vi "Update SequencerInfo.vi"(8 "error in (no error)":errorcluster, 10 "SequencerInfo":refnum<class "SequencerInfo.lvclass">, 11 "UI in":refnum<class "UI.lvclass">) -> (0 "error out":errorcluster, 3 "UI out":refnum<class "UI.lvclass">)   [LabVIEW 2015, in "UI.lvlib" / "UI.lvclass"]
uses:
  UI.lvclass
  Sequencer/SequencerInfo.lvclass
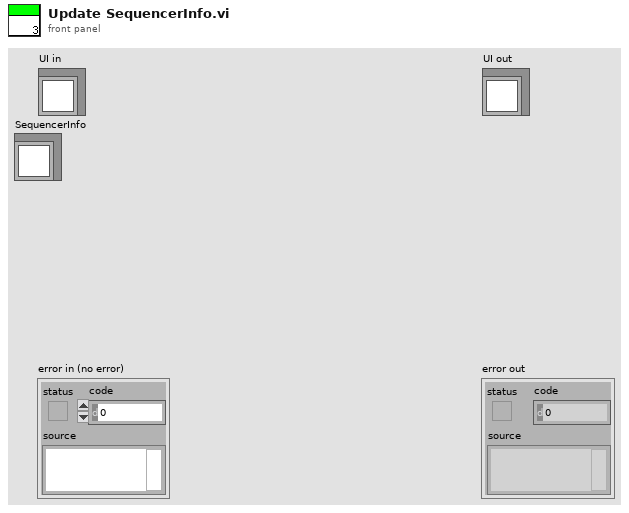
[diagram p1: front panel]
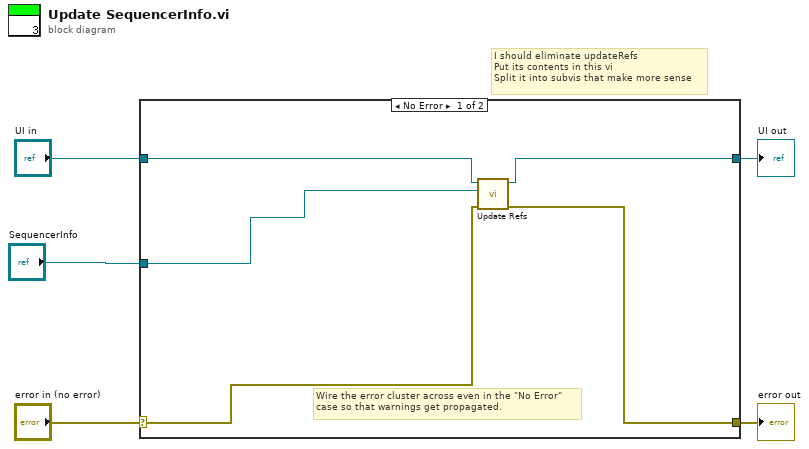
[diagram p0: block diagram]
diagram:
  # "I should eliminate updateRefs\nPut its contents in this vi\nSplit it into subvis that make more sense"
  n1 = case shown="No Error" "error in (no error)" {
    selector: "error in (no error)" -> [w9 w12]
    tunnel: [w8 w12] -> w4
    tunnel: [w10 w11] -> w2
    tunnel: "UI in" -> [w7 w11]
    tunnel: "SequencerInfo" -> [w6 _]
    frame No Error {
      # "Wire the error cluster across even in the \"No Error\"\ncase so that warnings get propagated."
      n2 = call "Update Refs.vi"("error in (no error)"=w9, "SequencerInfo"=w6, "UI in"=w7) -> ("error out"=w8:errorcluster, "UI out"=w10:refnum<class "UI.lvclass">)  [unwired: 7 in]
    }
    frame Error {
    }
  }
  "error out" <- w4
  "UI out" <- w2
